vi "list - get folder names.vi"(5 "extension filter":string, 6 "Numeric sort?":bool=TRUE, 7 "regular expression":string="\\s*(\\S*)\\s*", 11 "folder path":path) -> (0 "Array":string[](array[string]), 2 "OK":bool)   [LabVIEW 2015]
uses:
  <vilib>/regexp/Match Regular Expression.xnode
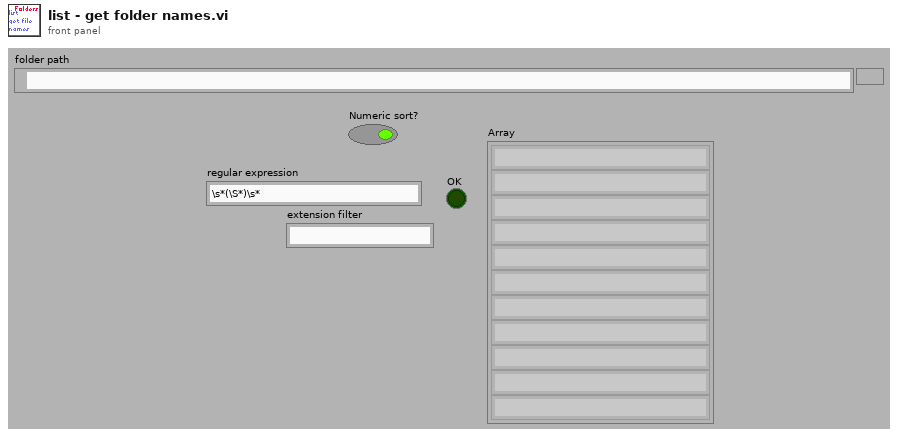
[diagram p1: front panel]
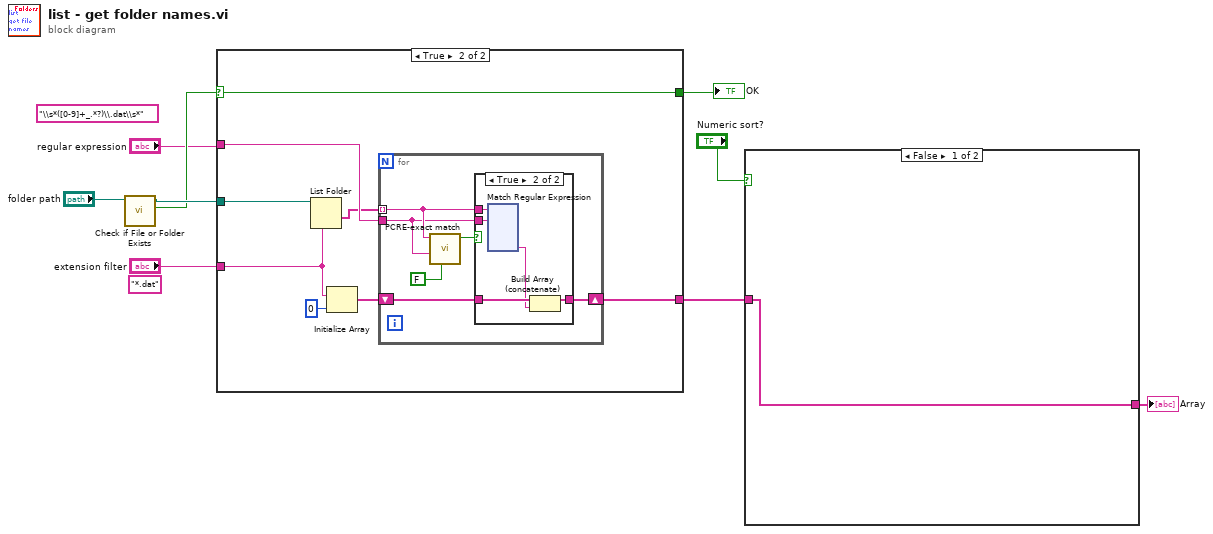
[diagram p0: block diagram]
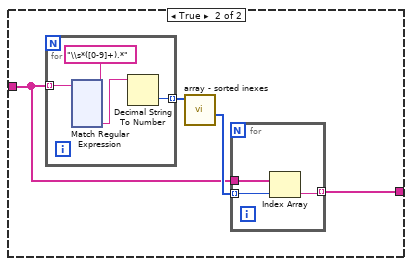
[diagram p2: hidden frame]
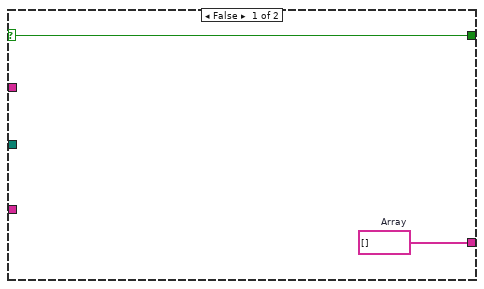
[diagram p3: hidden frame]
diagram:
  (unwired) "\\s*([0-9]+_.*?)\\.dat\\s*" ("regular expression")
  (unwired) "*.dat" ("pattern")
  n1 = call <vilib>:"Check if File or Folder Exists.vi"("path"="folder path") -> ("file or folder exists?"=w7:bool, "dup path"=w8:path)  [unwired: 8 in, 1 out]
  n2 = case shown="True" w7 {
    selector: w7 -> [w10 w13]
    tunnel: "extension filter" -> [_ w19]
    tunnel: "regular expression" -> [_ w16]
    tunnel: w8 -> [_ w15]
    tunnel: [w11 w14] -> w3
    tunnel: [w10 w13] -> w4
    frame False {
      w11 = string[] []  # Array
    }
    frame True {
      n3 = List Folder(path=w15, pattern=w19) -> (folder names=w12:string[])  [unwired: 2 in, 3 out]
      n4 = Initialize Array(w19, 0 ("dimension size")) -> (w17:string[])
      n5 = for {
        tunnel: w12 -> [w23] mode=indexing
        shift-right: [w24] -> w14
        shift-left: w17 -> [w25]
        tunnel: w16 -> [w21]
        n6 = call "PCRE-exact match.vi"("quote specials"=FALSE ("Boolean"), "regular expression"=w21, "input string"=w23) -> ("exact match"=w22:bool)  [unwired: 6 in, 2 out]
        n7 = case shown="True" w22 {
          tunnel: w21 -> [_ w31]
          tunnel: w25 -> [w26 w30]
          tunnel: [w26 w28] -> w24
          tunnel: w23 -> [_ w27]
          frame False {
          }
          frame True {
            n8 = xnode "Match Regular Expression"("input string"=w27, "regular expression"=w31) -> ("submatch 1"=w29:string)  [unwired: 4 in, 5 out]
            n9 = Build Array (concatenate)(w30, w29) -> (w28:string[])
          }
        }
      }
    }
  }
  "OK" <- w4
  n10 = case shown="False" "Numeric sort?" {
    tunnel: w3 -> [w145 w147]
    tunnel: [w145 w146] -> w2
    frame False {
    }
    frame True {
      n11 = for {
        tunnel: w147 -> [w156] mode=indexing
        tunnel: [w153] -> w149 mode=indexing
        n12 = xnode "Match Regular Expression"("input string"=w156, "regular expression"="\\s*([0-9]+).*") -> ("submatch 1"=w154:string)  [unwired: 4 in, 5 out]
        n13 = Decimal String To Number(string=w154) -> (number=w153:i32)  [unwired: 2 in, 1 out]
      }
      n14 = call "array - sorted inexes.vi"("x"=w149) -> ("index array"=w148:i32[])  [unwired: 9 in, 1 out]
      n15 = for {
        tunnel: w148 -> [w152] mode=indexing
        tunnel: w147 -> [w151]
        tunnel: [w150] -> w146 mode=indexing
        n16 = Index Array(array=w151, index=w152) -> (element=w150:string)
      }
    }
  }
  "Array" <- w2
